vi "layout.vi"(0 "reference":refnum<class "AbstractNode.lvclass">, 1 "graph":refnum<class "Graph.lvclass">, 2 "graphics":refnum<class "Graphics.lvclass">, 3 "grid":refnum<class "Grid.lvclass">, 5 "error in (no error)":errorcluster) -> (14 "reference out":refnum<class "AbstractNode.lvclass">, 19 "error out":errorcluster)   [LabVIEW 2014, in "AbstractNode.lvclass"]
doc: "public void layout(Graph g, Graphics2D g2, Grid grid)"
uses:
  <resource>/Framework/Providers/Open_GDS/UML/AbstractNode_class/AbstractNode.lvclass
  <resource>/Framework/Providers/Open_GDS/UML/Grid_class/Grid.lvclass
  <resource>/Framework/Providers/Open_GDS/UML/Graphics_class/Graphics.lvclass
  <resource>/Framework/Providers/Open_GDS/UML/Graph_class/Graph.lvclass
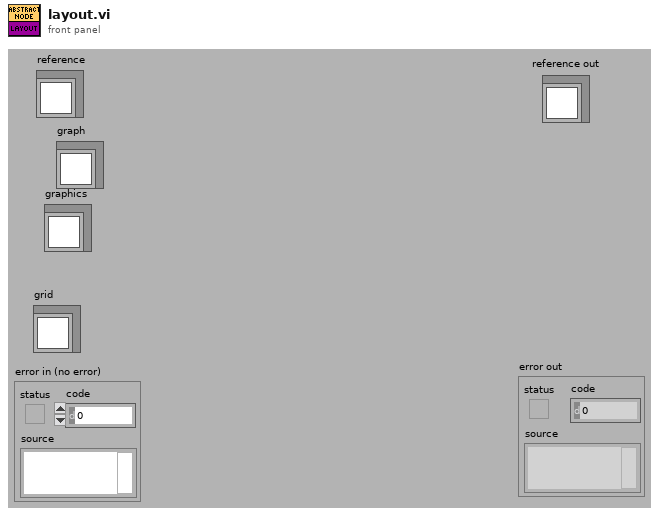
[diagram p1: front panel]
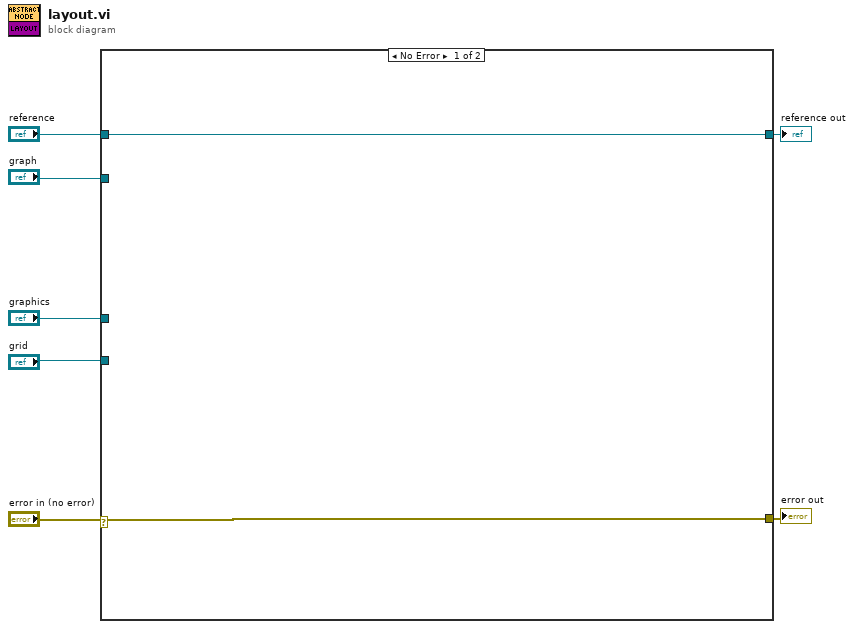
[diagram p0: block diagram]
diagram:
  n1 = case shown="No Error" "error in (no error)" {
    selector: "error in (no error)" -> [w8 w10]
    tunnel: "reference" -> [w9 w11]
    tunnel: [w8 w10] -> w6
    tunnel: [w9 w11] -> w5
    tunnel: "graph" -> [_ _]
    tunnel: "graphics" -> [_ _]
    tunnel: "grid" -> [_ _]
    frame No Error {
    }
    frame Error {
    }
  }
  "reference out" <- w5
  "error out" <- w6
